vi "Shut Down Device.vi"(8 "error in (no error)":errorcluster, 11 "Laser Quantum in":refnum<class "Laser.lvclass">) -> (0 "error out":errorcluster, 3 "Laser Quantum out":refnum<class "Laser.lvclass">)   [LabVIEW 2018, in "Laser.lvlib" / "Laser.lvclass"]
uses:
  Laser.lvclass
  Laser.lvclass/Laser.ctl
  Device/Device.lvclass
  Laser.lvlib
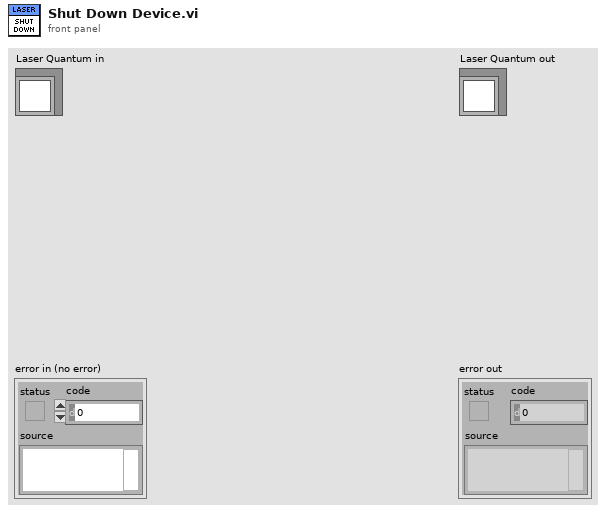
[diagram p1: front panel]
types:
  T1 = typedef "Laser Configuration.ctl" = cluster{"Serial Port":refnum<visa-resource-name>, "Laser Type":enum16{"Disable", "Laser Quantum", "Coherent OBIS", "PRM1-Z8", "Coherent HOPS"}, "Polarizer Amplitude":dbl, "Polarizer Theta Zero":dbl, "Wavelength":u16}
  T2 = enum16{"Disable", "Laser Quantum", "Coherent OBIS", "PRM1-Z8", "Coherent HOPS"}
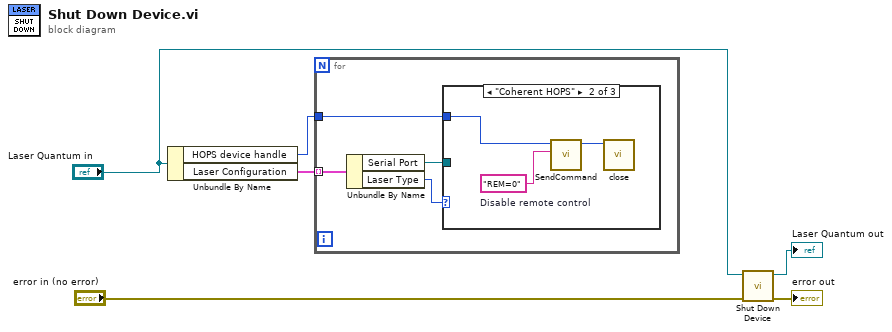
[diagram p0: block diagram]
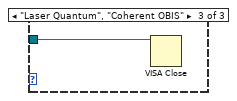
[diagram p3: hidden frame]
diagram:
  n1 = Unbundle By Name("Laser Quantum in") -> ("HOPS device handle"=w1:u64, "Laser Configuration"=w2:T1[])
  n2 = for {
    tunnel: w2 -> [w10] mode=indexing
    tunnel: w1 -> [w7]
    n3 = Unbundle By Name(w10) -> ("Serial Port"=w9:refnum<visa-resource-name>, "Laser Type"=w8:T2)
    n4 = case shown="\"Coherent HOPS\"" w8 {
      tunnel: w9 -> [_ _ w14]
      tunnel: w7 -> [_ w12 _]
      frame "Disable", Default {
      }
      frame "Coherent HOPS" {
        w13 = "REM=0"  # Disable remote control
        n5 = call "SendCommand.vi"("Command"=w13, "Device Handle"=w12) -> ("Dup Handle"=w11:u64)  [unwired: 4 in, 3 out]
        n6 = call "close.vi"("Device Handle"=w11) -> ()  [unwired: 8 in, 1 out]
      }
      frame "Laser Quantum", "Coherent OBIS" {
        n7 = VISA Close(VISA resource name=w14) -> ()  [unwired: 1 in, 1 out]
      }
    }
  }
  n8 = call-parent "Shut Down Device.vi"("error in (no error)"="error in (no error)", "Device in"="Laser Quantum in") -> ("error out"=→"error out":errorcluster, "Device out"=→"Laser Quantum out":refnum<class "Laser.lvclass">)  [unwired: 8 in]
